vi "calibrateSafeState.vi"(8 "error in (no error)":errorcluster, 11 "Channel in":refnum<class "Channel.lvclass">) -> (0 "error out":errorcluster, 2 "calibratedValue":dbl, 3 "Channel out":refnum<class "Channel.lvclass">)   [LabVIEW 2011, in "Tools.lvlib" / "DatabaseHelpers.lvlib" / "Channel.lvclass"]
uses:
  Channel.lvclass
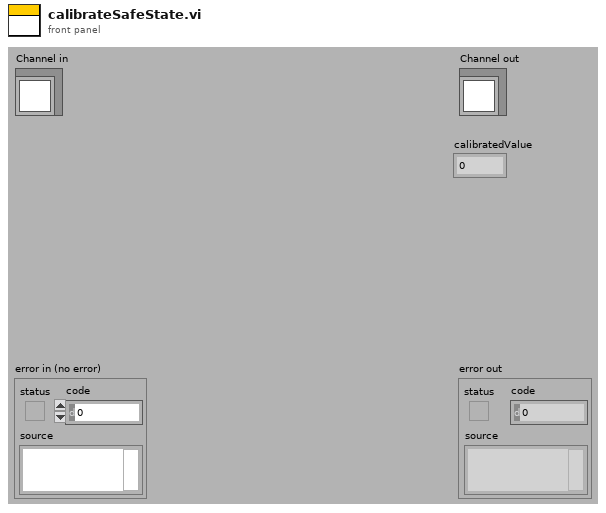
[diagram p1: front panel]
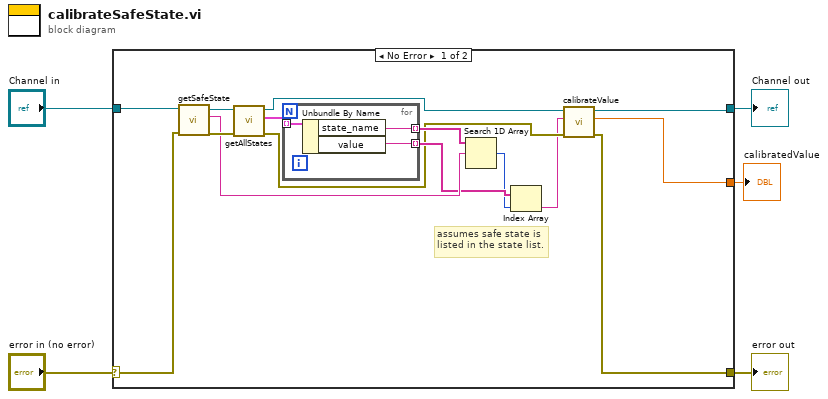
[diagram p0: block diagram]
diagram:
  n1 = case shown="No Error" "error in (no error)" {
    selector: "error in (no error)" -> [w6 w25]
    tunnel: [w7 w25] -> w4
    tunnel: [w8 w24] -> w2
    tunnel: "Channel in" -> [w10 w24]
    tunnel: [w9 _] -> w1
    frame No Error {
      # "assumes safe state is\nlisted in the state list."
      n2 = call "getSafeState.vi"("error in (no error)"=w6, "Channel.lvclass in"=w10) -> ("error out"=w19:errorcluster, "safe_state"=w16:string, "Channel.lvclass out"=w20:refnum<class "Channel.lvclass">)  [unwired: 7 in]
      n3 = call "getAllStates.vi"("error in (no error)"=w19, "Channel.lvclass in"=w20) -> ("error out"=w12:errorcluster, "states"=w18:cluster{"state_name":string, "value":string}[], "Channel.lvclass out"=w13:refnum<class "Channel.lvclass">)  [unwired: 7 in]
      n4 = for {
        tunnel: w18 -> [w23] mode=indexing
        tunnel: [w22] -> w17 mode=indexing
        tunnel: [w21] -> w15 mode=indexing
        n5 = Unbundle By Name(w23) -> ("state_name"=w22:string, "value"=w21:string)
      }
      n6 = Search 1D Array(1D array=w17, element=w16) -> (index of element=w14:i32)  [unwired: 1 in]
      n7 = Index Array(array=w15, index=w14) -> (element=w11:string)
      n8 = call-dynamic "calibrateValue.vi"("error in (no error)"=w12, "value"=w11, "Channel in"=w13) -> ("error out"=w7:errorcluster, "calibratedValue"=w9:dbl, "Channel out"=w8:refnum<class "Channel.lvclass">)  [unwired: 6 in]
    }
    frame Error {
    }
  }
  "error out" <- w4
  "Channel out" <- w2
  "calibratedValue" <- w1
